vi "Read Rotronic.vi"(8 "error in":errorcluster, 11 "tCRD Data in":refnum<class "tCRD Data.lvclass">) -> (0 "error out":errorcluster, 2 "Rotronic":cluster{"RH":sgl, "T":sgl}, 3 "tCRD Data out":refnum<class "tCRD Data.lvclass">)   [LabVIEW 2015, in "tCRD Data.lvclass"]
uses:
  tCRD Data.lvclass
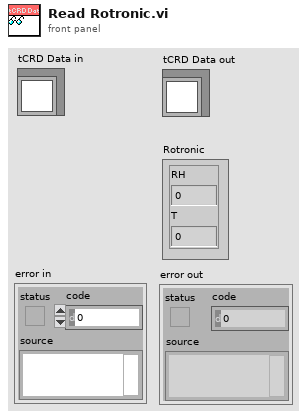
[diagram p1: front panel]
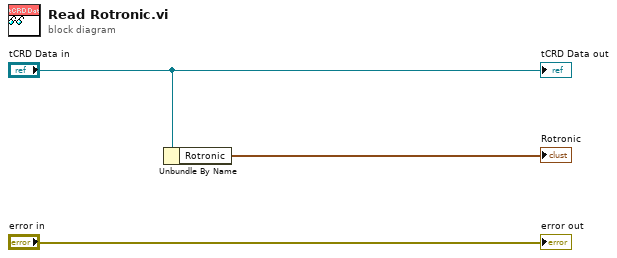
[diagram p0: block diagram]
diagram:
  n1 = Unbundle By Name("tCRD Data in") -> ("Rotronic"=→"Rotronic":cluster{"RH":sgl, "T":sgl})
  "error out" <- "error in"
  "tCRD Data out" <- "tCRD Data in"
